vi "solar_voy Launch.vi"(6 "Suppress Errors? (T)":bool=TRUE, 8 "error in (no error)":errorcluster, 9 "Open FP? (F)":bool, 10 "Ports":T1[](array[typedef]), 11 "Voyager Refnum in":T3) -> (0 "error out":errorcluster, 3 "Voyager Refnum out":T3)   [LabVIEW 2018]
doc: "This launches a TCP read process for each port. If the port does not exist, no process is launched."
uses:
  solar_voy_ctl TCP.ctl
  solar_voy_ctl Port Setup.ctl
  solar_voy_ctl Voyager Refnum.ctl
  solar_voy_ctl Port.ctl
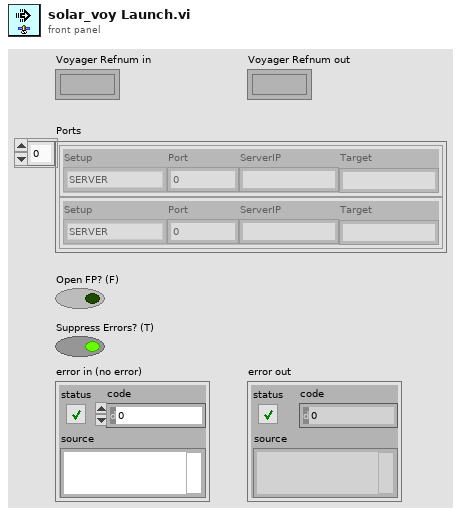
[diagram p1: front panel]
types:
  T1 = typedef "solar_voy_ctl Port.ctl" = cluster{"Setup":T2, "Port":u16, "ServerIP":string, "Target":string}
  T2 = typedef "solar_voy_ctl Port Setup.ctl" = enum8{"SERVER", "CLIENT", "SERVER_CMD", "SERVER_TLM"}
  T3 = typedef "solar_voy_ctl Voyager Refnum.ctl" = refnum<k1>
  T4 = typedef "solar_voy_ctl Voyager.ctl" = cluster{"PACKETS":T5[], "COSMOS_Root":path, "CMD_HDR":T10, "TLM_HDR":T10, "TCPs":T11[], "VoyagerIDOffset":cluster{"VoyagerIDOffset":u16[], "Target Names":string[]}}
  T5 = typedef "solar_voy_def_ctl PACKET.ctl" = cluster{"PACKET_ID":T6, "ENDIAN":enum8{"BIG", "LITTLE"}, "DESC":string, "HZRD":bool, "ITEMS":T7[], "NoExport":bool, "last_time":timestamp, "last_count":u32, "last_data":string}
  T6 = typedef "solar_voy_def_ctl PACKET_ID.ctl" = cluster{"ID":u16, "CMD":enum8{"CMD", "TLM"}, "TARGET":string, "PACKET":string}
  T7 = typedef "solar_voy_def_ctl ITEM.ctl" = cluster{"NAME":string, "OFFSET":i32, "SIZE":i32, "TYPE":T8, "EACH_SIZE":i32, "LVTYPE":T9, "MIN":dbl, "MAX":dbl, "DEFAULT":string, "DESC":string, "ID":bool, "MODIFIERS":variant, "last_value":variant}
  T8 = typedef "solar_voy_def_ctl ITEM TYPE.ctl" = enum8{"BLOCK", "INT", "UINT", "FLOAT", "STRING"}
  T9 = typedef "solar_type Item Type.ctl" = enum16{"NULL", "UNKNOWN", "CLUSTER", "I8", "I16", "I32", "I64", "U8", "U16", "U32", "U64", "U8_ENUM", "U16_ENUM", "U32_ENUM", "SGL", "DBL", "BOOLEAN", "STRING", "PATH", "VISA", "TAG", "TIME", "I8_1D", "I16_1D", "I32_1D", "I64_1D", "U8_1D", "U16_1D", "U32_1D", "U64_1D", "U8_ENUM_1D", "U16_ENUM_1D", "U32_ENUM_1D", "SGL_1D", "DBL_1D", "BOOLEAN_1D", "STRING_1D", "PATH_1D", "VISA_1D", "TAG_1D", "TIME_1D", "I8_2D", "I16_2D", "I32_2D", "I64_2D", "U8_2D", "U16_2D", "U32_2D", "U64_2D", "U8_ENUM_2D", "U16_ENUM_2D", "U32_ENUM_2D", "SGL_2D", "DBL_2D", "BOOLEAN_2D", "STRING_2D", "PATH_2D", "VISA_2D", "TAG_2D", "TIME_2D"}
  T10 = typedef "solar_voy_def_ctl HDR.ctl" = cluster{"ITEMS":T7[], "LENGTH_NAME":string, "LENGTH_VALUE_OFFSET":i32, "ID_NAME":string, "ENDIAN":enum8{"BIG", "LITTLE"}, "GUID_NAME":string, "DEFAULT_TARGET":string, "DEFAULT_PACKET":string, "DEFAULT_ERROR":string}
  T11 = typedef "solar_voy_ctl TCP.ctl" = cluster{"Connected":bool, "Port":u16, "Listener":refnum<k5>, "ServerIP":string, "TCP":refnum<k5>, "Setup":T2, "VIRefnum":refnum<vi>, "TARGETS_CMD":string[], "TARGETS_TLM":string[]}
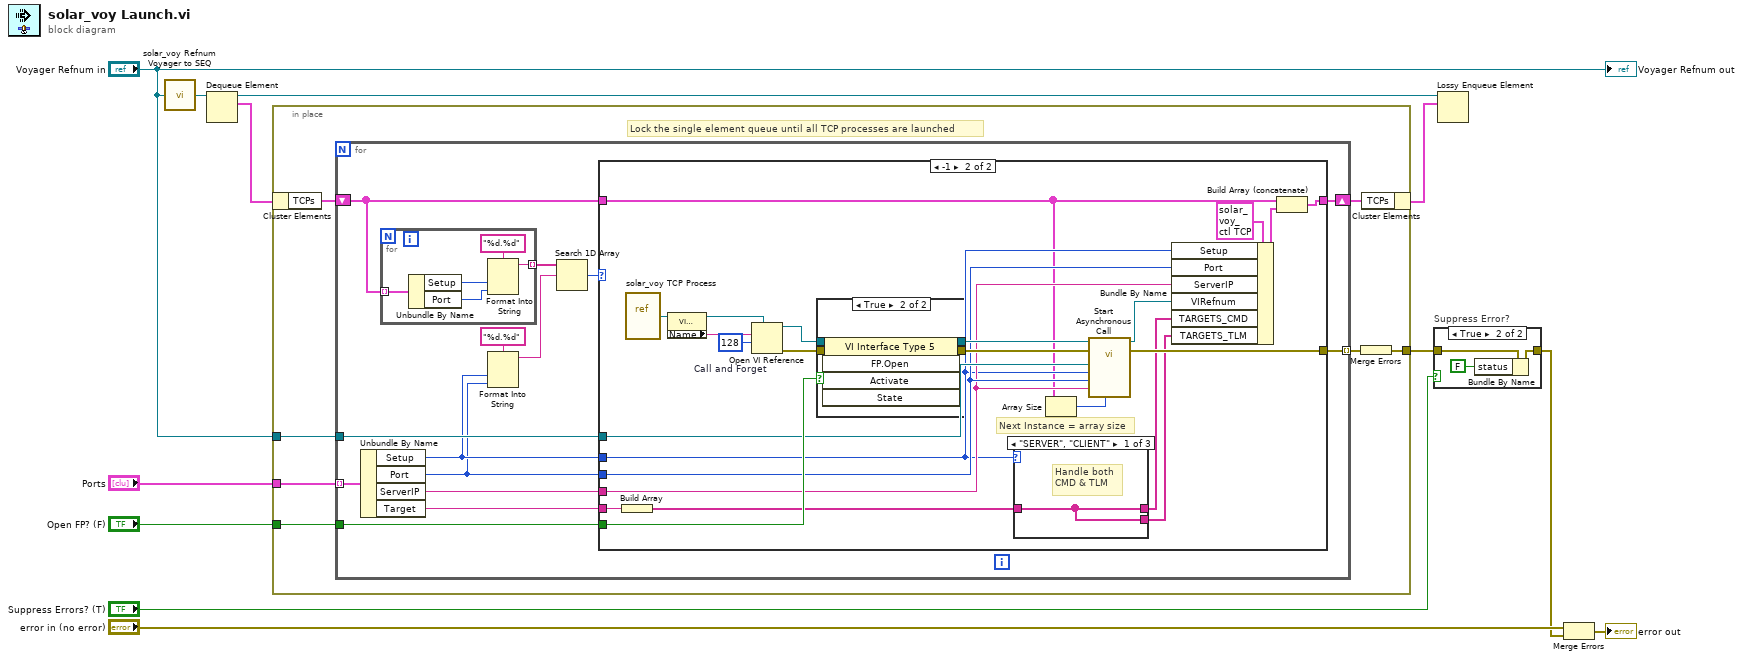
[diagram p0: block diagram]
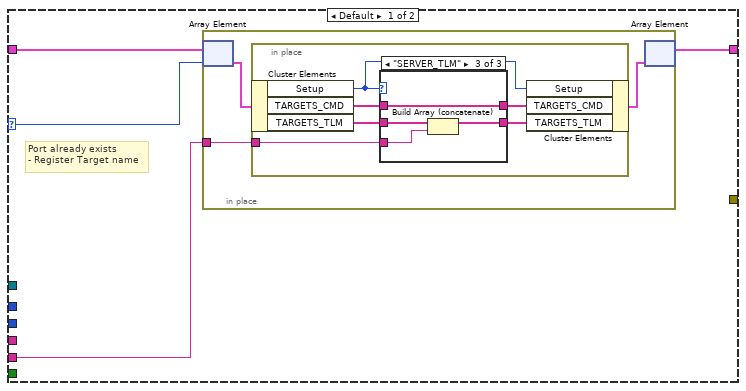
[diagram p2: hidden frame]
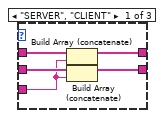
[diagram p3: hidden frame]
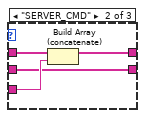
[diagram p4: hidden frame]
diagram:
  n1 = call "solar_voy Refnum Voyager to SEQ.vi"("Voyager Refnum"="Voyager Refnum in") -> ("Voyager SEQ"=w3:refnum<queue>)
  n2 = Dequeue Element(queue=w3) -> (queue out=w8:refnum<queue>, element=w2:T4)  [unwired: 2 in, 2 out]
  n3 = in-place {
    in-place-border: [w13] -> w7
    in-place-border: "Open FP? (F)" -> [w18]
    in-place-border: "Voyager Refnum in" -> [w17]
    in-place-border: "Ports" -> [w16]
    # "Lock the single element queue until all TCP processes are launched"
    n4 = in-place-cluster #1(w2) -> ("TCPs"=w15:T11[])
    n5 = for {
      tunnel: [w33] -> w19 mode=indexing
      tunnel: w18 -> [w32]
      tunnel: w17 -> [w31]
      tunnel: w16 -> [w30] mode=indexing
      shift-right: [w28] -> w14
      shift-left: w15 -> [w27]
      n6 = Unbundle By Name(w30) -> ("Setup"=w24:T2, "Port"=w23:u16, "ServerIP"=w29:string, "Target"=w20:string)
      n7 = for {
        tunnel: w27 -> [w38] mode=indexing
        tunnel: [w34] -> w26 mode=indexing
        n8 = Unbundle By Name(w38) -> ("Setup"=w37:T2, "Port"=w36:u16)
        n9 = Format Into String(format string="%d.%d", w37, w36) -> (resulting string=w34:string)  [unwired: 2 in, 1 out]
      }
      n10 = Format Into String(format string="%d.%d", w24, w23) -> (resulting string=w22:string)  [unwired: 2 in, 1 out]
      n11 = Search 1D Array(1D array=w26, element=w22) -> (index of element=w21:i32)  [unwired: 1 in]
      n12 = case shown="-1" w21 {
        selector: w21 -> [w40 _]
        tunnel: [_ w80] -> w33
        tunnel: w32 -> [_ w79]
        tunnel: w31 -> [_ w78]
        tunnel: w23 -> [_ w74]
        tunnel: w24 -> [_ w71]
        tunnel: w29 -> [_ w73]
        tunnel: [w41 w72] -> w28
        tunnel: w27 -> [w42 w66]
        tunnel: w20 -> [w39 w70]
        frame Default {
          # "Port already exists\n- Register Target name"
          n13 = in-place {
            in-place-border: w39 -> [w43]
            n14 = in-place-array #2(w42, w40) -> (w45:T11)
            n15 = in-place {
              in-place-border: w43 -> [w49]
              n16 = in-place-cluster #3(w45) -> ("Setup"=w46:T2, "TARGETS_CMD"=w51:string[], "TARGETS_TLM"=w47:string[])
              n17 = case shown="\"SERVER_TLM\"" w46 {
                tunnel: w51 -> [w56 w60 w63]
                tunnel: [w54 w59 w63] -> w50
                tunnel: w49 -> [w52 w58 w61]
                tunnel: [w53 w57 w62] -> w48
                tunnel: w47 -> [w55 w57 w64]
                frame "SERVER", "CLIENT" {
                  n18 = Build Array (concatenate)(w56, w52) -> (w54:string[])
                  n19 = Build Array (concatenate)(w55, w52) -> (w53:string[])
                }
                frame "SERVER_CMD" {
                  n20 = Build Array (concatenate)(w60, w58) -> (w59:string[])
                }
                frame "SERVER_TLM" {
                  n21 = Build Array (concatenate)(w64, w61) -> (w62:string[])
                }
              }
              n22 = in-place-cluster #3("Setup"=w46, "TARGETS_CMD"=w50, "TARGETS_TLM"=w48) -> (w44:T11)
            }
            n23 = in-place-array #2(w44) -> (w41:T11[])  [unwired: 1 out]
          }
        }
        frame -1 {
          w85 = 128  # Call and Forget
          # "Next Instance = array size"
          n24 = Build Array(w70) -> (w69:string[])
          n25 = vi-ref "solar_voy TCP Process.vi"() -> (w88:refnum<vi>)
          n26 = property class="VI (strict)"(reference=w88) -> (reference out=w86:refnum<vi>, "Name"=w87:string)  [unwired: 1 in, 1 out]
          n27 = Open VI Reference(type specifier VI Refnum (for type only)=w86, vi path=w87, options=w85) -> (vi reference=w82:refnum<vi>, error out=w84:errorcluster)  [unwired: 3 in]
          n28 = case shown="True" w79 {
            tunnel: w84 -> [w93 w97]
            tunnel: [w93 w96] -> w83
            tunnel: w82 -> [w92 w95]
            tunnel: [w92 w94] -> w81
            frame False {
            }
            frame True {
              n29 = invoke class="VI Interface Type 5" method="FP.Open"(reference=w95, error in=w97) -> (reference out=w94:refnum<vi>, error out=w96:errorcluster)  [unwired: 3 in, 3 out]
            }
          }
          n30 = case shown="\"SERVER\", \"CLIENT\"" w71 {
            tunnel: w69 -> [w89 w90 w91]
            tunnel: [w89 w90 _] -> w68
            tunnel: [w89 _ w91] -> w67
            frame "SERVER", "CLIENT" {
              # "Handle both\nCMD & TLM"
            }
            frame "SERVER_CMD" {
              # "Handle CMD\n(inbound) only"
            }
            frame "SERVER_TLM" {
              # "Handle TLM\n(outbound) only"
            }
          }
          n31 = Array Size(array=w66) -> (size(s)=w65:i32)
          n32 = call-by-ref "Start Asynchronous Call"(reference=w81, error in=w83, "Instance"=w65, "IP Address"=w73, "Port"=w74, "Setup"=w71, "Voyager Refnum"=w78) -> (reference out=w76:refnum<vi>, error out=w80:errorcluster)  [unwired: 7 in]
          n33 = Bundle By Name(cluster=T11 {"Connected"=FALSE, "Port"=0, "Listener"=refnum, "ServerIP"="", "TCP"=refnum, "Setup"=enum."SERVER", "VIRefnum"=refnum, "TARGETS_CMD"=[], "TARGETS_TLM"=[]} ("TCP"), "Setup"=w71, "Port"=w74, "ServerIP"=w73, "VIRefnum"=w76, "TARGETS_CMD"=w68, "TARGETS_TLM"=w67) -> (w75:T11)
          n34 = Build Array (concatenate)(w66, w75) -> (w72:T11[])
        }
      }
    }
    n35 = Merge Errors(w19) -> (w13:errorcluster)
    n36 = in-place-cluster #1("TCPs"=w14) -> (w1:T4)
  }
  n37 = case "Suppress Error?" shown="True" "Suppress Errors? (T)" {
    tunnel: w7 -> [w98 w101]
    tunnel: [w98 w100] -> w10
    frame False {
    }
    frame True {
      n38 = Bundle By Name(cluster=w101, "status"=FALSE) -> (w100:errorcluster)
    }
  }
  n39 = Lossy Enqueue Element(queue=w8, element=w1) -> ()  [unwired: 1 in, 4 out]
  n40 = Merge Errors("error in (no error)", w10) -> (→"error out":errorcluster)
  "Voyager Refnum out" <- "Voyager Refnum in"
